vi "MVE Bitfield Value Picker.vi"(10 "Item Path":string, 11 "Bitfield in":string) -> (3 "Bitfield Out":string)   [LabVIEW 2016]
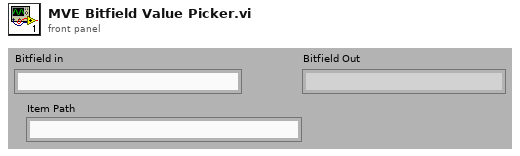
[diagram p1: front panel]
types:
  T1 = enum16{"Scaling Invert Mask", "Scaling Select Mask", "Alarm Invert Mask", "Alarm Select Mask", "Initial Value"}
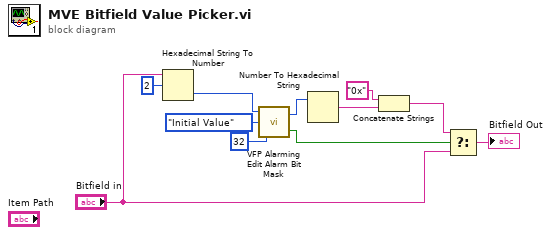
[diagram p0: block diagram]
diagram:
  n1 = Hexadecimal String To Number(string="Bitfield in", offset=2) -> (number=w6:u32)  [unwired: 1 in, 1 out]
  n2 = call <resource>:"VFP Alarming Edit Alarm Bit Mask.vi"("Max Length"=32, "Mask Type"=T1."Initial Value", "Mask Hex Display"=w6) -> ("Update"=w8:bool, "Mask Out"=w5:u32)
  n3 = Number To Hexadecimal String(2:w5) -> (0:w4:string)  [unwired: 1 in]
  n4 = Concatenate Strings("0x" ("string"), w4) -> (w3:string)
  n5 = Select(t=w3, s=w8, f="Bitfield in") -> (s? t:f=→"Bitfield Out":string)
